vi "Set Shutter Index.vi"(0 "Notifier Name In":string, 7 "Shutter Index":u8, 11 "Error In":errorcluster) -> (4 "Notifier Name Out":string, 15 "Error Out":errorcluster)   [LabVIEW 2020]
uses:
  Microscopes Type Defs/Microscope Notifier.ctl
  Microscopes Type Defs/Microscope Actions.ctl
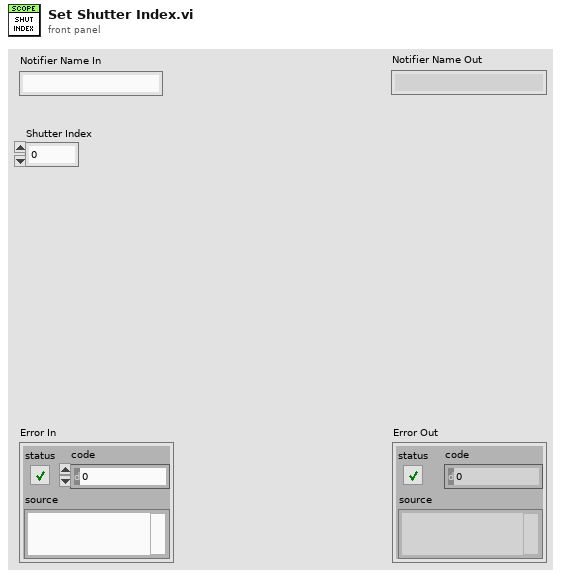
[diagram p1: front panel]
types:
  T1 = typedef "Microscope Notifier.ctl" = cluster{"Actions":T2, "Action Done":bool, "Objective Index":u8, "Objective Z Position (um)":dbl, "Lamp Index":u8, "Lamp State":bool, "Output Port":u8, "Shutter Index":u8, "Shutter State":bool, "Dichroic Wheel Position":u8, "Parameter":string, "Parameter Value":string, "Base Locked?":bool, "Obj Speed":u32, "Obj Acceleration":u32, "Obj Deceleration":u32, "Lamp Power (%)":dbl}
  T2 = typedef "Microscope Actions.ctl" = enum16{"Do Nothing", "Lock Base", "Unlock Base", "Get Objective Index", "Get Objective Z Position", "Get Lamp State", "Get Lamp Power", "Get Output Port", "Get Shutter State", "Get Dichroic Wheel Position", "Set Lamp Index", "Set Shutter Index", "Set Objective Z Position", "Set Lamp State", "Set Lamp Power", "Set Output Port", "Set Shutter State", "Set Dichroic Wheel Position", "Set Objective", "Abort Move", "Set Parameter", "Get Parameter", "Quit"}
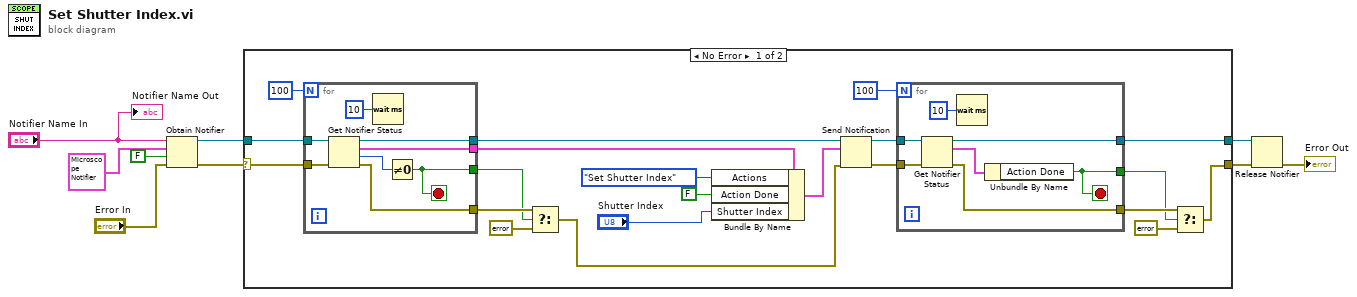
[diagram p0: block diagram]
diagram:
  n1 = Obtain Notifier(name (unnamed)="Notifier Name In", notification data type=T1 {"Actions"=enum."Get Objective Index", "Action Done"=FALSE, "Objective Index"=0, "Objective Z Position (um)"=0.0, "Lamp Index"=0, "Lamp State"=FALSE, "Output Port"=0, "Shutter Index"=0, "Shutter State"=FALSE, "Dichroic Wheel Position"=0, "Parameter"="", "Parameter Value"="", "Base Locked?"=FALSE, "Obj Speed"=0, "Obj Acceleration"=0, "Obj Deceleration"=0, "Lamp Power (%)"=0.0} ("Microscope Notifier"), create if not found? (T)=FALSE, error in (no error)="Error In") -> (notifier out=w6:refnum<notifier>, error out=w7:errorcluster)  [unwired: 1 out]
  n2 = case shown="No Error" w7 {
    selector: w7 -> [w28 w47]
    tunnel: w6 -> [w30 w46]
    tunnel: [w19 w47] -> w2
    tunnel: [w20 w46] -> w3
    frame No Error {
      n3 = for {
        N: 100 -> [_]
        tunnel: w30 -> [w45]
        tunnel: [w43] -> w16
        tunnel: [w41] -> w26
        tunnel: w28 -> [w40]
        tunnel: [w39] -> w17
        tunnel: [w38] -> w27
        stop <- w43 stop-if-true
        n4 = Get Notifier Status(notifier=w45, error in (no error)=w40) -> (notifier out=w41:refnum<notifier>, current notification=w38:T1, # waiting=w44:i32, error out=w39:errorcluster)  [unwired: 1 out]
        n5 = Wait (ms)(milliseconds to wait=u32 10) -> ()  [unwired: 1 out]
        n6 = Not Equal To 0?(x=w44) -> (x != 0?=w43:bool)
      }
      n7 = Select(t=w17, s=w16, f=errorcluster {"status"=TRUE, "code"=0, "source"="IX81 Base Error: Base busy time out."}) -> (s? t:f=w14:errorcluster)
      n8 = Bundle By Name(cluster=w27, "Actions"=Microscope_Actions."Set Shutter Index", "Action Done"=FALSE, "Shutter Index"="Shutter Index") -> (w25:T1)
      n9 = Send Notification(notification=w25, notifier=w26, error in (no error)=w14) -> (notifier out=w21:refnum<notifier>, error out=w24:errorcluster)
      n10 = for {
        N: 100 -> [_]
        tunnel: w21 -> [w37]
        tunnel: [w35] -> w20
        tunnel: w24 -> [w34]
        tunnel: [w33] -> w12
        tunnel: [w31] -> w11
        stop <- w31 stop-if-true
        n11 = Get Notifier Status(notifier=w37, error in (no error)=w34) -> (notifier out=w35:refnum<notifier>, current notification=w32:T1, error out=w33:errorcluster)  [unwired: 2 out]
        n12 = Wait (ms)(milliseconds to wait=u32 10) -> ()  [unwired: 1 out]
        n13 = Unbundle By Name(w32) -> ("Action Done"=w31:bool)
      }
      n14 = Select(t=w12, s=w11, f=errorcluster {"status"=TRUE, "code"=0, "source"="IX81 Base Error: Action didn't complete."}) -> (s? t:f=w19:errorcluster)
    }
    frame Error {
    }
  }
  n15 = Release Notifier(notifier=w3, error in (no error)=w2) -> (error out=→"Error Out":errorcluster)  [unwired: 1 in, 2 out]
  "Notifier Name Out" <- "Notifier Name In"
